vi "TestFT.vi"() -> ()   [LabVIEW 2010]
panel:
  out "Fz":bool
  out "Tr":bool
  out "Tz":dbl(knob) scale=-10.0..10.0
  out "Ty":dbl(knob) scale=-10.0..10.0
  out "Tx":dbl(knob) scale=-10.0..10.0
  out "Fz":dbl(knob) scale=-10.0..10.0
  out "Fy":dbl(knob) scale=-10.0..10.0
  out "Fx":dbl(knob) scale=-10.0..10.0
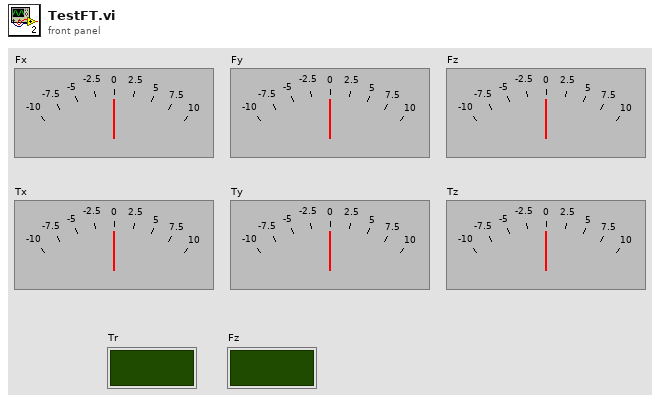
[diagram p1: front panel]
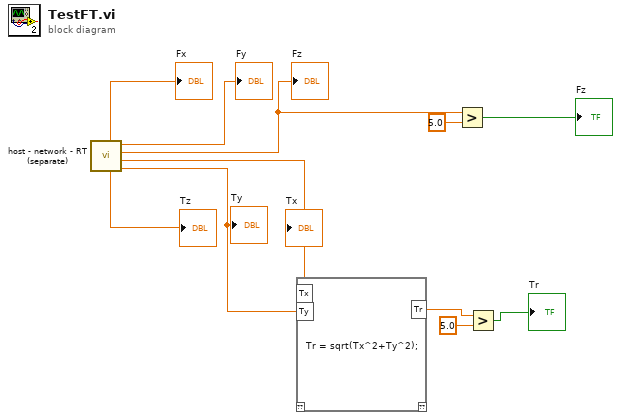
[diagram p0: block diagram]
diagram:
  n1 = call "host - network - RT (separate).vi"() -> ("Fx"=→"Fx":dbl, "Tz"=→"Tz":dbl, "Fy"=→"Fy":dbl, "Fz"=w8:dbl, "Tx"=w4:dbl, "Ty"=w5:dbl)  [unwired: 1 in]
  "Fz" <- w8
  "Tx" <- w4
  "Ty" <- w5
  n2 = script code="Tr = sqrt(Tx^2+Ty^2);"("Tx"=w4, "Ty"=w5) -> ("Tr"=w2:dbl)  [unwired: 1 in, 1 out]
  n3 = Greater?(x=w8, y=5.0) -> (0:→"Fz":bool)
  n4 = Greater?(x=w2, y=5.0) -> (0:→"Tr":bool)
